vi "Matrix to a Power.vi"() -> ()   [LabVIEW 2023]
doc: "The following example shows the matrix power function defined using diagonalization. If a matrix is symmetric or invertible, it is diagonalizable. This decomposition takes the form P*D*P^-1 where D is a diagonal matrix whose elements are the eigenvalues and P is the matrix of eigenvectors as columns.\n\nIf A is diagonalizable, then:\nA^n = (P*D*P^-1)^n = (P*D*P^-1)(P*D*P^-1)... = P*(D^n)*P^-1.\n\nSince D is a diagonal matrix, D^n is just the diagonal elements to the nth power."
uses:
  <vilib>/Analysis/Matrix/Datatypes/RealMatrix.ctl
  <vilib>/Analysis/_algsub.llb/Real Matrix Norm.vi
  <vilib>/Analysis/baseanly.llb/Real Dot Product.vi
  <vilib>/Analysis/baseanly.llb/Real Inverse Matrix.vi
  <vilib>/Analysis/7linalg.llb/Create Special Real Matrix.vi
  <vilib>/Analysis/Matrix/Numeric/Multiply/Multiply - R,RM.vi
  <vilib>/Analysis/Matrix/Numeric/Subtract/Subtract - RM,RM.vi
  <vilib>/Analysis/Matrix/Numeric/Absolute Value/Absolute Value - RM.vi
  <vilib>/Analysis/7linalg.llb/Real Eigenvalues and Vectors.vi
  <vilib>/Analysis/7linalg.llb/Create Special Complex Matrix.vi
  <vilib>/Analysis/baseanly.llb/Complex Inverse Matrix.vi
  <vilib>/Analysis/Matrix/Numeric/Multiply/Multiply - CM,CM.vi
  <vilib>/Analysis/Matrix/Numeric/Conversions/Matrix To Array - CM.vi
  <vilib>/Analysis/Matrix/Numeric/Conversions/Array To Matrix - RA2.vi
  <vilib>/Analysis/Matrix/Numeric/Add/Add - RM,RM.vi
  <vilib>/Analysis/Matrix/Numeric/Multiply/Multiply - RM,R.vi
  <vilib>/Analysis/Matrix/Numeric/Complex/Complex To Cartesian - CM.vi
  <vilib>/Analysis/Matrix/Numeric/Multiply/Multiply - RM,RM.vi
  <vilib>/Analysis/Matrix/NI_Matrix.lvlib
  <vilib>/Analysis/NI_AALPro.lvlib
  <vilib>/Analysis/NI_AALBase.lvlib
panel:
  in  "Stop":bool
  out "A^n":T1
  in  "Matrix Power n":i32=3
  in  "Real Matrix A":T1=[[-1.0, 2.0], [1.0, 3.0]]
  # "Overview: Demonstrates the use of the Linear Algebra VIs to raise a matrix to a specified power.\nRequirements: LabVIEW Full Development System\nInstructions:\n1. Run the VI.\n2. Modify the Real Matrix A and Matrix Power n values, and view the results in the A^n output matrix.\n3. Click Stop to stop the VI."
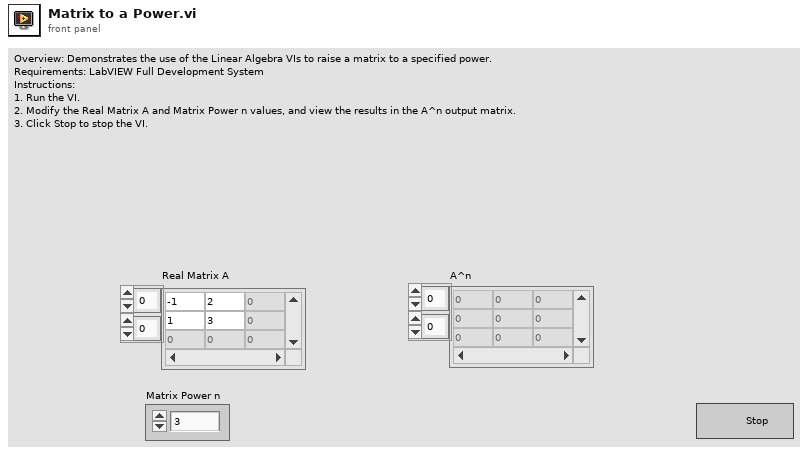
[diagram p1: front panel]
types:
  T1 = typedef "NI_Matrix.lvlib/RealMatrix.ctl" = dbl[][]
  T2 = typedef "NI_Matrix.lvlib/ComplexMatrix.ctl" = cdb[][]
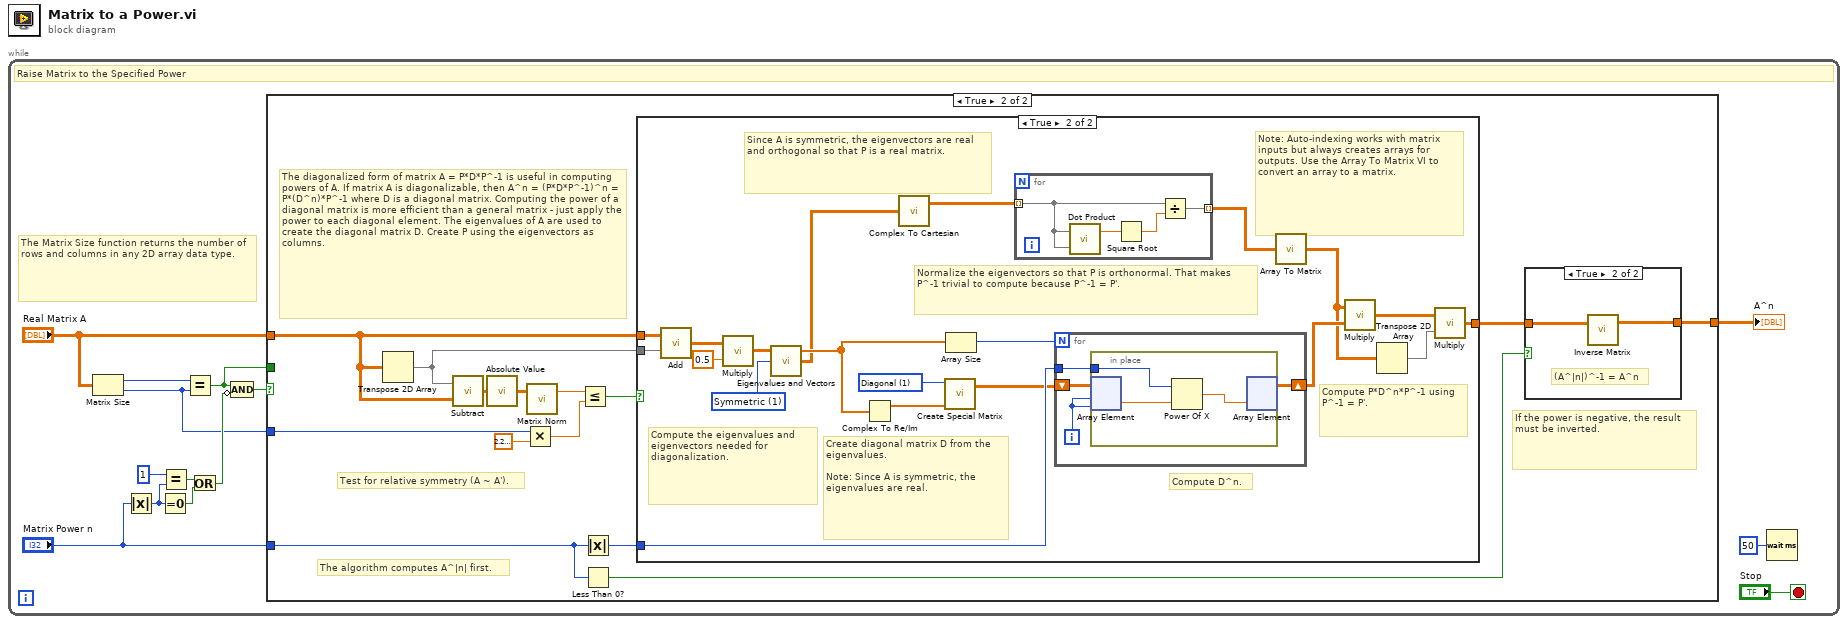
[diagram p0: block diagram]
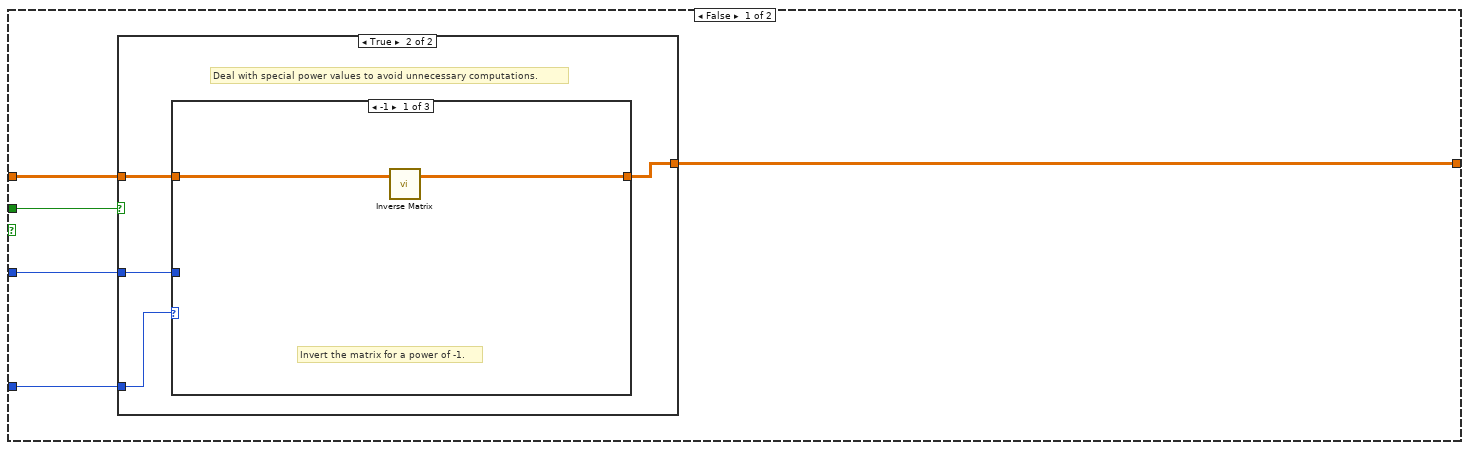
[diagram p2: hidden frame]
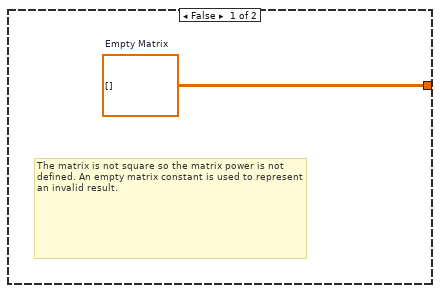
[diagram p3: hidden frame]
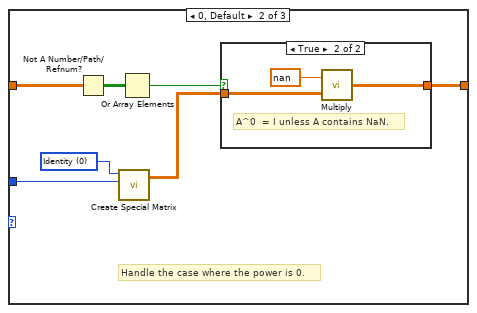
[diagram p4: hidden frame]
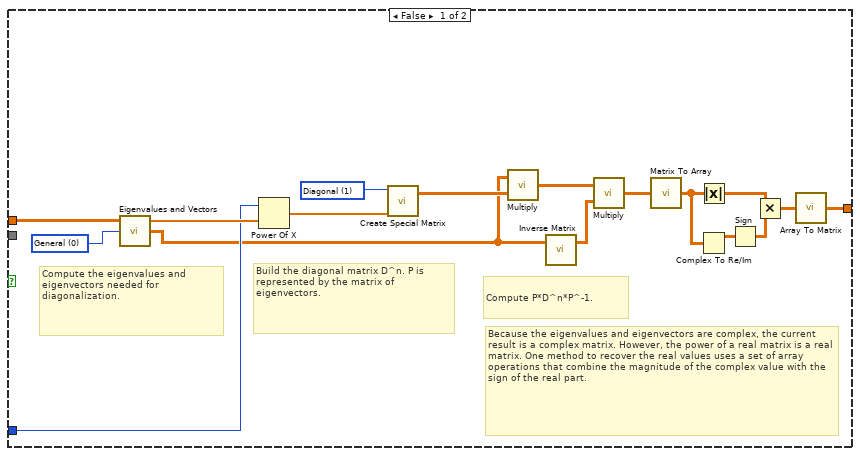
[diagram p8: hidden frame]
diagram:
  n1 = while {
    stop <- "Stop" stop-if-true
    # "The Matrix Size function returns the number of rows and columns in any 2D array data type."
    # "Raise Matrix to the Specified Power"
    n2 = Matrix Size(0:"Real Matrix A") -> (1:w2:i32, 2:w1:i32)
    n3 = Absolute Value(x="Matrix Power n") -> (abs(x)=w5:i32)
    n4 = Equal To 0?(x=w5) -> (x = 0?=w7:bool)
    n5 = Equal?(x=1, y=w5) -> (x = y?=w8:bool)
    n6 = Equal?(x=w2, y=w1) -> (x = y?=w4:bool)
    n7 = Or(x=w8, y=w7) -> (x .or. y?=w6:bool)
    n8 = Compound Arithmetic op=AND(w4, invert w6) -> (w11:bool)
    n9 = case shown="True" w11 {
      tunnel: "Real Matrix A" -> [w15 w39]
      tunnel: w1 -> [w16 w49]
      tunnel: "Matrix Power n" -> [w17 w44]
      tunnel: [w18 w41] -> w14
      tunnel: w4 -> [w19 _]
      frame False {
        n10 = case shown="True" w19 {
          tunnel: [w20 w22] -> w18
          tunnel: w17 -> [_ w24]
          tunnel: w16 -> [_ w23]
          tunnel: w15 -> [_ w21]
          frame False {
            w20 = T1 []  # Empty Matrix
            # "The matrix is not square so the matrix power is not defined. An empty matrix constant is used to represent an invalid result."
          }
          frame True {
            # "Deal with special power values to avoid unnecessary computations."
            n11 = case shown="-1" w24 {
              tunnel: w23 -> [_ w33 _]
              tunnel: [w26 w28 w38] -> w22
              tunnel: w21 -> [w25 w32 w38]
              frame -1 {
                # "Invert the matrix for a power of -1."
                n12 = call-poly <vilib>:"Inverse Matrix.vi"("Input Matrix"=w25) -> ("Inverse Matrix"=w26:T1)  [unwired: 1 in, 1 out]
              }
              frame 0, Default {
                w27 = 0 items=["Identity", "Diagonal", "Toeplitz", "Vandermonde", "Companion", "Hankel", "Hadamard", "Wilkinson", "Hilbert", "Inverse Hilbert", "Rosser", "Pascal"] ("matrix type")
                # "Handle the case where the power is 0."
                n13 = Not A Number/Path/Refnum?(number/path/refnum=w32) -> (NaN/Path/Refnum?=w31:bool[][])
                n14 = call-poly <vilib>:"Create Special Matrix.vi"("matrix type"=w27, "matrix size"=w33) -> ("Special Matrix"=w29:T1)  [unwired: 2 in, 2 out]
                n15 = Or Array Elements(Boolean array=w31) -> (logical OR=w30:bool)
                n16 = case shown="True" w30 {
                  tunnel: w29 -> [w34 w37]
                  tunnel: [w34 w35] -> w28
                  frame False {
                  }
                  frame True {
                    # "A^0  = I unless A contains NaN."
                    n17 = call-poly <vilib>:"Multiply.vi"("Real Matrix A"=w37, "Real Scalar c"=nan) -> ("c * A"=w35:T1)
                  }
                }
              }
              frame 1 {
                # "No work is needed for a power of 1."
              }
            }
          }
        }
      }
      frame True {
        # "The diagonalized form of matrix A = P*D*P^-1 is useful in computing powers of A. If matrix A is diagonalizable, then A^n = (P*D*P^-1)^n = P*(D^n)*P^-1 where D is a diagonal matrix. Computing the power of a diagonal matrix is more efficient than a general matrix - just apply the power to each diagonal element. The eigenvalues of A are used to create the diagonal matrix D. Create P using the eigenvectors as columns."
        # "If the power is negative, the result must be inverted."
        # "The algorithm computes A^|n| first."
        # "Test for relative symmetry (A ~ A')."
        n18 = Transpose 2D Array(2D array=w39) -> (transposed array=w40:T1)
        n19 = call-poly <vilib>:"Subtract.vi"("Real Matrix B"=w39, "Real Matrix A"=w40) -> ("A - B"=w52:T1)
        n20 = call-poly <vilib>:"Absolute Value.vi"("Real Matrix A"=w52) -> ("|A|"=w51:T1)
        n21 = Multiply(x=w49, y=2.220446049250313e-16) -> (x*y=w46:dbl)
        n22 = call-poly <vilib>:"Matrix Norm.vi"("Input Matrix"=w51) -> ("norm"=w47:dbl)  [unwired: 1 in, 1 out]
        n23 = Less Or Equal?(x=w47, y=w46) -> (x <= y?=w48:bool)
        n24 = Absolute Value(x=w44) -> (abs(x)=w45:i32)
        n25 = Less Than 0?(x=w44) -> (x < 0?=w42:bool)
        n26 = case shown="True" w48 {
          tunnel: w39 -> [w72 w91]
          tunnel: w40 -> [_ w92]
          tunnel: w45 -> [w70 w82]
          tunnel: [w60 w85] -> w43
          frame False {
            w56 = 1 items=["Identity", "Diagonal", "Toeplitz", "Vandermonde", "Companion", "Hankel", "Hadamard", "Wilkinson", "Hilbert", "Inverse Hilbert", "Rosser", "Pascal"] ("matrix type")
            w57 = 0 items=["General", "Symmetric"] ("matrix type")
            # "Because the eigenvalues and eigenvectors are complex, the current result is a complex matrix. However, the power of a real matrix is a real matrix. One method to recover the real values uses a set of array operations that combine the magnitude of the complex value with the sign of the real part."
            # "Compute P*D^n*P^-1."
            # "Build the diagonal matrix D^n. P is represented by the matrix of eigenvectors."
            # "Compute the eigenvalues and eigenvectors needed for diagonalization."
            n27 = call-poly <vilib>:"Eigenvalues and Vectors.vi"("matrix type"=w57, "Input Matrix"=w72) -> ("Eigenvectors"=w67:T2, "Eigenvalues"=w71:cdb[])  [unwired: 1 in, 1 out]
            n28 = Power Of X(1:w71, 2:w70) -> (0:w69:cdb[])
            n29 = call-poly <vilib>:"Create Special Matrix.vi"("matrix type"=w56, "Input Vector1"=w69) -> ("Special Matrix"=w68:T2)  [unwired: 2 in, 2 out]
            n30 = call-poly <vilib>:"Multiply.vi"("Complex Matrix B"=w68, "Complex Matrix A"=w67) -> ("A * B"=w66:T2)
            n31 = call-poly <vilib>:"Inverse Matrix.vi"("Input Matrix"=w67) -> ("Inverse Matrix"=w65:T2)  [unwired: 1 in, 1 out]
            n32 = call-poly <vilib>:"Multiply.vi"("Complex Matrix B"=w65, "Complex Matrix A"=w66) -> ("A * B"=w62:T2)
            n33 = call-poly <vilib>:"Matrix To Array.vi"("Complex Matrix"=w62) -> ("Complex 2D Array"=w59:cdb[][])
            n34 = Absolute Value ("Absolute Value.vi")(x=w59) -> (abs(x)=w61:dbl[][])
            n35 = Complex To Re/Im ("Complex To Cartesian.vi")(x + iy=w59) -> (x=w64:dbl[][])  [unwired: 1 out]
            n36 = Sign(1:w64) -> (0:w63:dbl[][])
            n37 = Multiply ("Multiply.vi")(x=w61, y=w63) -> (x*y=w58:dbl[][])
            n38 = call-poly <vilib>:"Array To Matrix.vi"("Real 2D Array"=w58) -> ("Real Matrix"=w60:T1)
          }
          frame True {
            w73 = 1 items=["Identity", "Diagonal", "Toeplitz", "Vandermonde", "Companion", "Hankel", "Hadamard", "Wilkinson", "Hilbert", "Inverse Hilbert", "Rosser", "Pascal"] ("matrix type")
            w81 = 1 items=["General", "Symmetric"] ("matrix type")
            # "Compute D^n."
            # "Create diagonal matrix D from the eigenvalues.\n\nNote: Since A is symmetric, the eigenvalues are real."
            # "Note: Auto-indexing works with matrix inputs but always creates arrays for outputs. Use the Array To Matrix VI to convert an array to a matrix."
            # "Normalize the eigenvectors so that P is orthonormal. That makes P^-1 trivial to compute because P^-1 = P'."
            # "Since A is symmetric, the eigenvectors are real and orthogonal so that P is a real matrix."
            # "Compute P*D^n*P^-1 using P^-1 = P'."
            # "Compute the eigenvalues and eigenvectors needed for diagonalization."
            n39 = call-poly <vilib>:"Add.vi"("Real Matrix B"=w92, "Real Matrix A"=w91) -> ("A + B"=w90:T1)
            n40 = call-poly <vilib>:"Multiply.vi"("Real Scalar c"=0.5 ("x*y"), "Real Matrix A"=w90) -> ("A * c"=w88:T1)
            n41 = call-poly <vilib>:"Eigenvalues and Vectors.vi"("matrix type"=w81, "Input Matrix"=w88) -> ("Eigenvectors"=w77:T2, "Eigenvalues"=w83:cdb[])  [unwired: 1 in, 1 out]
            n42 = Complex To Re/Im ("Complex To Cartesian.vi")(x + iy=w83) -> (x=w74:dbl[])  [unwired: 1 out]
            n43 = call-poly <vilib>:"Complex To Cartesian.vi"("Complex Matrix R + Ii"=w77) -> ("Real Matrix R"=w79:T1)  [unwired: 1 out]
            n44 = call-poly <vilib>:"Create Special Matrix.vi"("matrix type"=w73, "Input Vector1"=w74) -> ("Special Matrix"=w76:T1)  [unwired: 2 in, 2 out]
            n45 = Array Size(array=w83) -> (size(s)=w75:i32)
            n46 = for {
              tunnel: w79 -> [w100] mode=indexing
              tunnel: [w101] -> w80 mode=indexing
              n47 = call-poly <vilib>:"Dot Product.vi"("Y Vector"=w100, "X Vector"=w100) -> ("X * Y"=w103:dbl)  [unwired: 1 out]
              n48 = Square Root(x=w103) -> (sqrt(x)=w102:dbl)
              n49 = Divide(x=w100, y=w102) -> (x/y=w101:dbl[])
            }
            n50 = for {
              N: w75 -> [_]
              shift-right: [w94] -> w84
              shift-left: w76 -> [w95]
              tunnel: w82 -> [w96]
              i -> [w93]
              n51 = in-place {
                in-place-border: w96 -> [w97]
                n52 = in-place-array #1(w95, w93, w93) -> (w99:dbl)
                n53 = Power Of X(1:w99, 2:w97) -> (0:w98:dbl)
                n54 = in-place-array #1(w98) -> (w94:T1)  [unwired: 2 out]
              }
            }
            n55 = call-poly <vilib>:"Array To Matrix.vi"("Real 2D Array"=w80) -> ("Real Matrix"=w78:T1)
            n56 = call-poly <vilib>:"Multiply.vi"("Real Matrix B"=w84, "Real Matrix A"=w78) -> ("A * B"=w87:T1)
            n57 = Transpose 2D Array(2D array=w78) -> (transposed array=w86:T1)
            n58 = call-poly <vilib>:"Multiply.vi"("Real Matrix B"=w86, "Real Matrix A"=w87) -> ("A * B"=w85:T1)
          }
        }
        n59 = case shown="True" w42 {
          tunnel: w43 -> [w53 w55]
          tunnel: [w53 w54] -> w41
          frame False {
            # "A^|n|=A^n"
          }
          frame True {
            # "(A^|n|)^-1 = A^n"
            n60 = call-poly <vilib>:"Inverse Matrix.vi"("Input Matrix"=w55) -> ("Inverse Matrix"=w54:T1)  [unwired: 1 in, 1 out]
          }
        }
      }
    }
    "A^n" <- w14
    n61 = Wait (ms)(milliseconds to wait=u32 50) -> ()  [unwired: 1 out]
  }
